vi "Read Condition.vi"(11 "Interlock Deny in":refnum<class "IL I32 Seize.lvclass">) -> (2 "Deny":i32[](array[numeric]), 3 "Interlock Deny out":refnum<class "IL I32 Seize.lvclass">)   [LabVIEW 2015, in "Interlocks.lvlib" / "IL I32 Seize.lvclass"]
uses:
  IL I32 Seize.lvclass
  IL I32 Seize.lvclass/IL I32 Seize.ctl
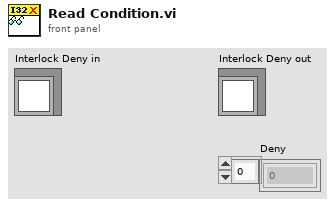
[diagram p1: front panel]
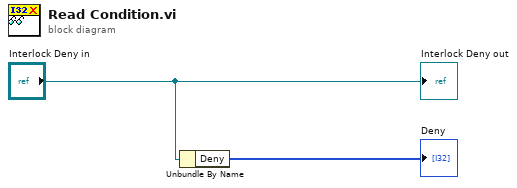
[diagram p0: block diagram]
diagram:
  n1 = Unbundle By Name("Interlock Deny in") -> ("Deny"=→"Deny":i32[])
  "Interlock Deny out" <- "Interlock Deny in"
